vi "BB_CameraDirectly from MJPG-Streamer.vi"(5 "remote port or service name":u16=5800, 7 "Operation":enum16{"Read", "Reopen", "Close"}(ring), 8 "error in":errorcluster, 9 "fps":i32=30, 10 "Image":T1, 11 "address":string="10.te.am.11") -> (0 "error out":errorcluster, 1 "Bandwidth (Mbps)":dbl=30.0, 2 "Image Out":T1, 3 "FPS":dbl)   [LabVIEW 2016]
doc: "This VI is intended for testing, examples, and demos. It assumes the camera is directly accssible from the computer and not the robot. It retrieves an image from either a USB or IP Axis camera.\n\nThis software is licensed. Open the labview\\readme\\WPI Robotics Library Open Source License.txt file for more information."
uses:
  <vilib>/vision/Image Controls.llb/IMAQ Image.ctl
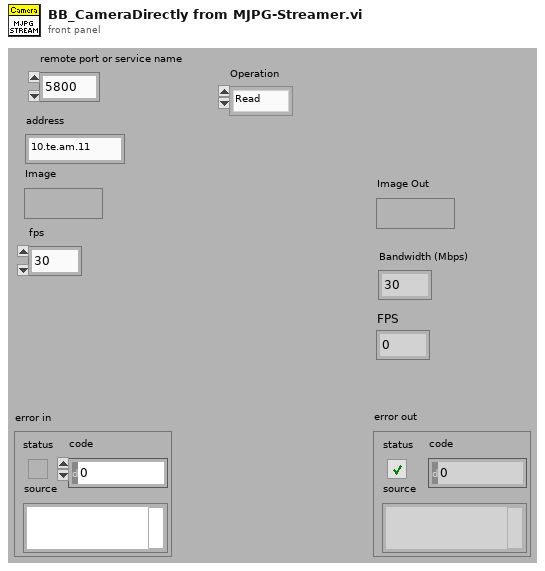
[diagram p1: front panel]
types:
  T1 = typedef "IMAQ Image.ctl" = refnum<image>
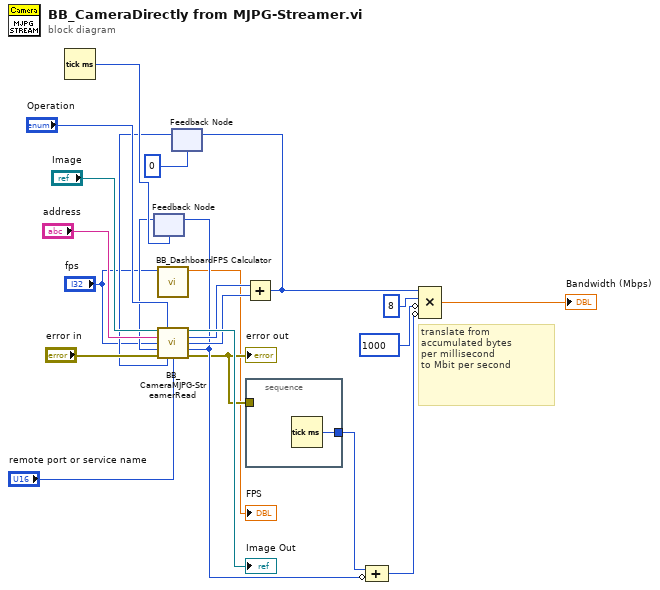
[diagram p0: block diagram]
diagram:
  # "translate from\naccumulated bytes\nper millisecond \nto Mbit per second"
  n1 = Tick Count (ms)() -> (millisecond timer value=w16:u32)
  n2 = feedback #1(w16) -> (w11:u32)
  n3 = call "BB_DashboardFPS Calculator.vi"("Average Count"="fps") -> ("fps"=→"FPS":dbl)  [unwired: 10 in]
  n4 = feedback #2(0) -> (w13:i32)
  n5 = call "BB_CameraMJPG-StreamerRead.vi"("Refnum in"="Image", "Operation"="Operation", "remote port or service name"="remote port or service name", "address"="address", "fps"="fps", "millisecond timer value in"=w11, "error in (no error)"="error in", "Numeric in"=w13) -> ("Refnum out"=→"Image Out":T1, "Numeric 3"=w9:i32, "Numeric out"=w12:i32, "millisecond timer value out"=w7:u32, "error out"=w6:errorcluster)  [unwired: 3 in]
  "error out" <- w6
  n6 = feedback-in #1(w7) -> ()
  n7 = Add(x=w9, y=w12) -> (x+y=w10:i32)
  n8 = feedback-in #2(w10) -> ()
  n9 = stacked-sequence {
    tunnel: [w23] -> w8
    tunnel: w6 -> [_]
    frame #0 {
      n10 = Tick Count (ms)() -> (millisecond timer value=w23:u32)
    }
  }
  n11 = Compound Arithmetic op=ADD(w8, invert w7) -> (w5:u32)
  n12 = Compound Arithmetic op=MULTIPLY(w10, 8 ("timeout ms (25000)"), invert 1000 ("timeout ms (25000)"), invert w5) -> (→"Bandwidth (Mbps)":dbl)
